vi "Set Waveforms.vi"(8 "error in (no error)":errorcluster, 10 "Waveforms":waveform(dbl)[](array[waveform]), 11 "Visualizer ID":T1) -> (0 "error out":errorcluster)   [LabVIEW 2016, in "Visualizer.lvlib"]
doc: "Put a waveform into the visualizer. If the visualizer has already been unpaused, this waveform will begin playing immediately."
uses:
  Visualizer.lvlib
  Visualizer Type ID.ctl
  Message.ctl
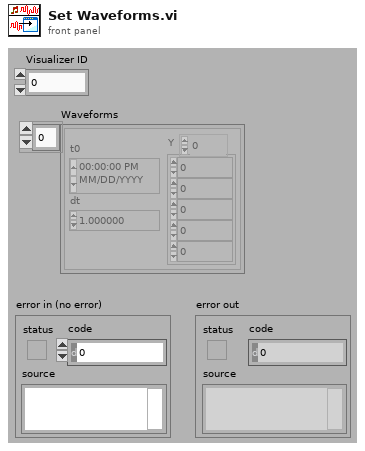
[diagram p1: front panel]
types:
  T1 = typedef "Visualizer.lvlib/Visualizer Type ID.ctl" = u32
  T2 = typedef "Visualizer.lvlib/Message.ctl" = cluster{"Command":string, "Data":variant}
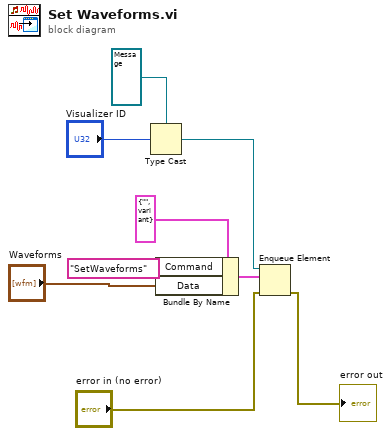
[diagram p0: block diagram]
diagram:
  n1 = Type Cast(type=refnum<queue> refnum ("queue out"), x="Visualizer ID") -> (*(type *) &x=w7:refnum<queue>)
  n2 = Bundle By Name(cluster=T2 {"Command"="", "Data"=variant} ("Message"), "Command"="SetWaveforms", "Data"="Waveforms") -> (w2:T2)
  n3 = Enqueue Element(queue=w7, element=w2, error in (no error)="error in (no error)") -> (error out=→"error out":errorcluster)  [unwired: 1 in, 2 out]
